vi "Manifold State.vi"(7 "Get/Set":enum16{"Get", "Set"}(ring), 8 "error in (no error)":errorcluster, 10 "New Port Statuses":map{i32, bool}(c390), 11 "FlexWorktable in":refnum<class "FlexWorktable.lvclass">) -> (0 "error out":errorcluster, 2 "Port Statuses":map{i32, bool}(c390), 3 "FlexWorktable out":refnum<class "FlexWorktable.lvclass">)   [LabVIEW 2024, in "FlexWorktable.lvclass"]
uses:
  FlexWorktable.lvclass
  FlexWorktable.lvclass/FlexWorktable.ctl
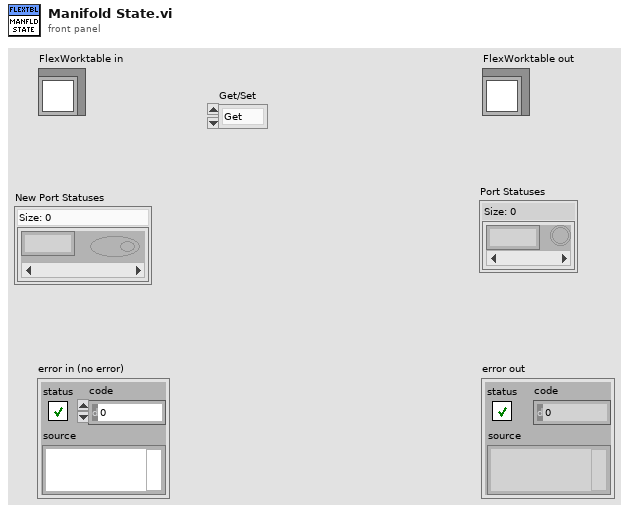
[diagram p1: front panel]
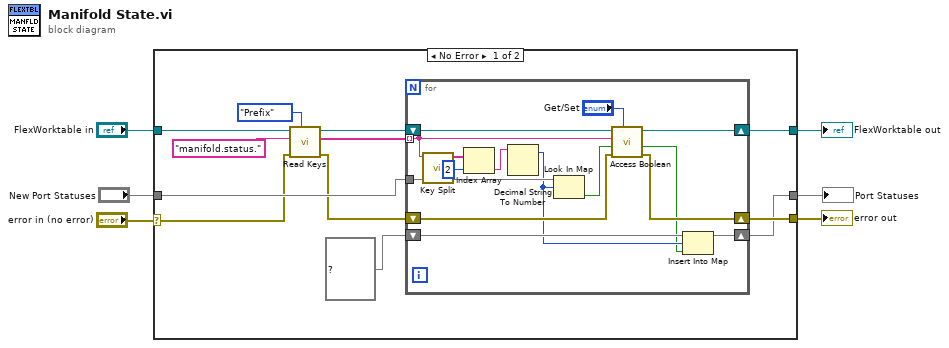
[diagram p0: block diagram]
diagram:
  n1 = case shown="No Error" "error in (no error)" {
    selector: "error in (no error)" -> [w14 w35]
    tunnel: [w12 w35] -> w5
    tunnel: [w11 w34] -> w3
    tunnel: "FlexWorktable in" -> [w17 w34]
    tunnel: "New Port Statuses" -> [w18 _]
    tunnel: [w7 _] -> w1
    frame No Error {
      n2 = call-dynamic "Read Keys.vi"("Prefix/Regex"=enum16{"Prefix", "Regex"}."Prefix", "error in (no error)"=w14, "Selector"="manifold.status.", "FlexWorktable in"=w17) -> ("error out"=w13:errorcluster, "Keys"=w9:string[], "FlexWorktable out"=w16:refnum<class "FlexWorktable.lvclass">)  [unwired: 5 in]
      n3 = for {
        tunnel: w18 -> [w28]
        shift-right: [w29] -> w12
        shift-left: w13 -> [w30]
        shift-right: [w32] -> w11
        shift-left: w16 -> [w33]
        tunnel: w9 -> [w27] mode=indexing
        shift-right: [w21] -> w7
        shift-left: map{i32, bool} {} ("Port Statuses 2") -> [w22]
        n4 = call "Key Split.vi"("Key"=w27) -> ("Key Elements"=w26:string[])  [unwired: 10 in]
        n5 = Index Array(array=w26, index=2) -> (element=w24:string)
        n6 = Decimal String To Number(string=w24) -> (offset past number=w20:i32)  [unwired: 2 in, 1 out]
        n7 = Look In Map(map=w28, key=w20) -> (value=w23:bool)  [unwired: 1 in, 1 out]
        n8 = call-dynamic "Access Boolean.vi"("Get/Set"="Get/Set", "error in (no error)"=w30, "Value in"=w23, "Key"=w27, "FlexWorktable in"=w33) -> ("error out"=w29:errorcluster, "Value out"=w19:bool, "FlexWorktable out"=w32:refnum<class "FlexWorktable.lvclass">)  [unwired: 4 in]
        n9 = Insert Into Map(map in=w22, key=w20, value=w19) -> (map out=w21:map{i32, bool})  [unwired: 2 out]
      }
    }
    frame Error {
    }
  }
  "error out" <- w5
  "FlexWorktable out" <- w3
  "Port Statuses" <- w1
